vi "Enum to List.vi"(8 "error in (no error)":errorcluster, 10 "Enum":variant) -> (0 "error out":errorcluster, 2 "Enum Strings":string[](array[string]))   [LabVIEW 2013, in "JKI_Python_Bridge_for_LV.lvlib" / "Call.lvclass"]
uses:
  Call.lvclass
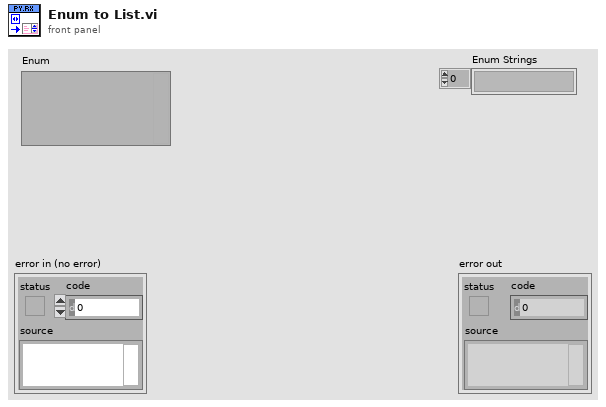
[diagram p1: front panel]
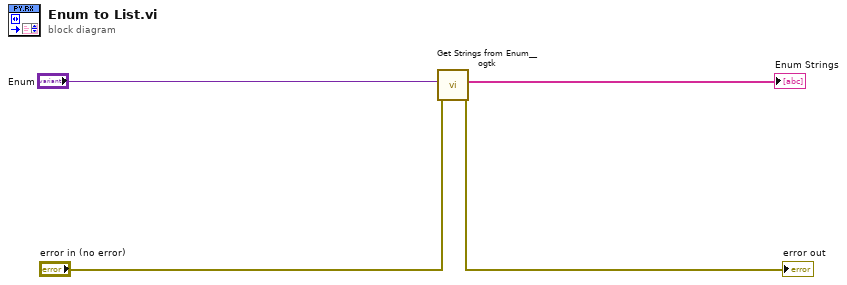
[diagram p0: block diagram]
diagram:
  n1 = call <userlib>:"Get Strings from Enum__ogtk.vi"("error in (no error)"="error in (no error)", "Enum"="Enum") -> ("error out"=→"error out":errorcluster, "Enum Strings"=→"Enum Strings":string[])  [unwired: 6 in, 2 out]
